vi "2D Array.vi"() -> ()   [LabVIEW 2020]
uses:
  <vilib>/DAQmx/read.llb/DAQmx Read (Analog 2D DBL NChan NSamp).vi
  <vilib>/DAQmx/create/channels.llb/DAQmx Create Channel (AI-Acceleration-Accelerometer).vi
  <vilib>/DAQmx/configure/timing.llb/DAQmx Timing (Sample Clock).vi
  <vilib>/DAQmx/miscellaneous.llb/DAQmx Fill In Error Info.vi
panel:
  out "subarray":dbl[](array[numeric])
  out "Acceleration Data - Graph":dbl[][](graph)
  out "Acceleration Data - Array":dbl[][](array[numeric])
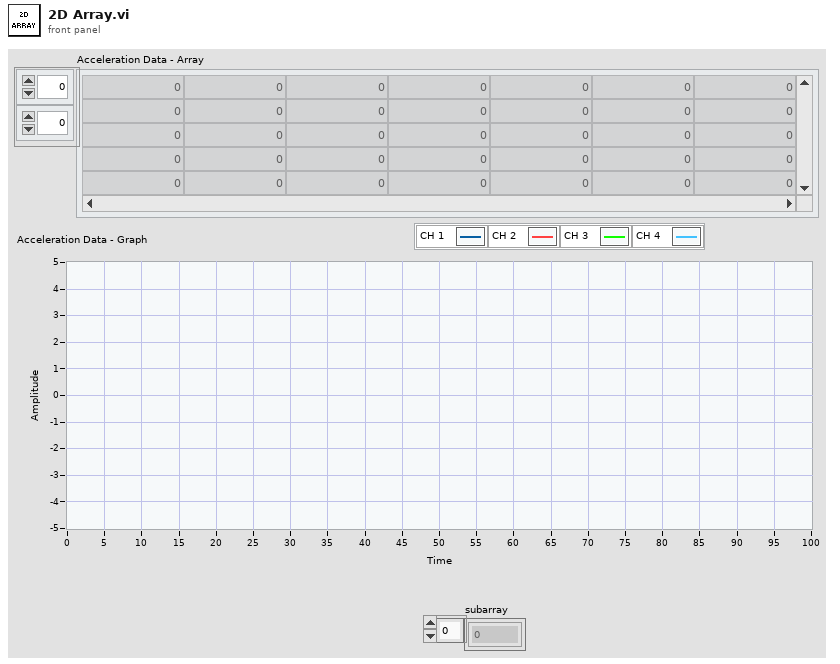
[diagram p1: front panel]
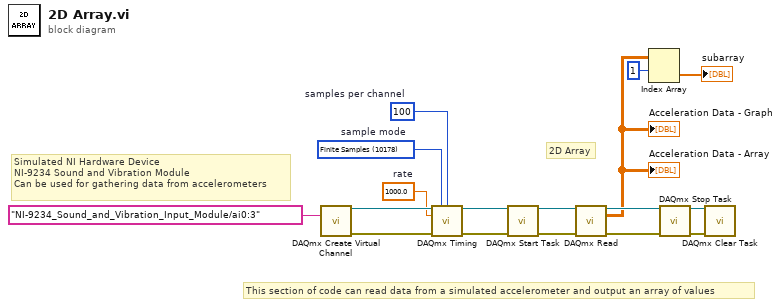
[diagram p0: block diagram]
diagram:
  w4 = 1000.0  # rate
  w5 = 100  # samples per channel
  w6 = 10178 items=["Finite Samples"=10178, "Continuous Samples"=10123, "Hardware Timed Single Point"=12522]  # sample mode
  # "2D Array"
  # "This section of code can read data from a simulated accelerometer and output an array of values"
  # "Simulated NI Hardware Device\nNI-9234 Sound and Vibration Module\nCan be used for gathering data from accelerometers"
  n1 = call-poly <vilib>:"DAQmx Create Virtual Channel.vi"("physical channels"=tag "NI-9234_Sound_and_Vibration_Input_Module/ai0:3") -> ("task out"=w10:refnum<k21>, "error out"=w9:errorcluster)  [unwired: 13 in]
  n2 = call-poly <vilib>:"DAQmx Timing.vi"("task/channels in"=w10, "sample mode"=w6, "samples per channel"=w5, "rate"=w4, "error in"=w9) -> ("task out"=w8:refnum<k21>, "error out"=w7:errorcluster)  [unwired: 9 in]
  n3 = call <vilib>:"DAQmx Start Task.vi"("task/channels in"=w8, "error in"=w7) -> ("task out"=w16:refnum<k21>, "error out"=w17:errorcluster)  [unwired: 12 in]
  n4 = call-poly <vilib>:"DAQmx Read.vi"("task/channels in"=w16, "error in"=w17) -> ("task out"=w14:refnum<k21>, "data"=w3:dbl[][], "error out"=w13:errorcluster)  [unwired: 11 in]
  "Acceleration Data - Array" <- w3
  "Acceleration Data - Graph" <- w3
  n5 = Index Array(array=w3, index (row)=1) -> (element=→"subarray":dbl[])  [unwired: 1 in]
  n6 = call <vilib>:"DAQmx Stop Task.vi"("task/channels in"=w14, "error in"=w13) -> ("task out"=w15:refnum<k21>, "error out"=w12:errorcluster)  [unwired: 12 in]
  n7 = call <vilib>:"DAQmx Clear Task.vi"("task in"=w15, "error in"=w12) -> ()  [unwired: 13 in, 1 out]
